vi "TrackingHelp.vi"() -> ()   [LabVIEW 2014]
panel:
  out "String":string="This mode is intended for tracking operation. Currently this mode works as a setpoint switcher where the ROV moves to the next WayPoint (WP) in the list when the current is reached. \n\nThe waypoint list will auto-index itself when entering new waypoints and is inserted automatically in the map view.\n\nIt is not possible to enter negative depth (height above the surface as ROVs cannot fly..yet).\n\nThe Generate Pattern Button opens a dialog box where inputs can be given in order to generate a lawn mower pattern. \n\nThe Read and Write WP buttons import and export the waypoints in their own file format: *.wp\n\nThe clear WP List button removes all the waypoints from the list, and also from the map."
  out "2D Picture":picture
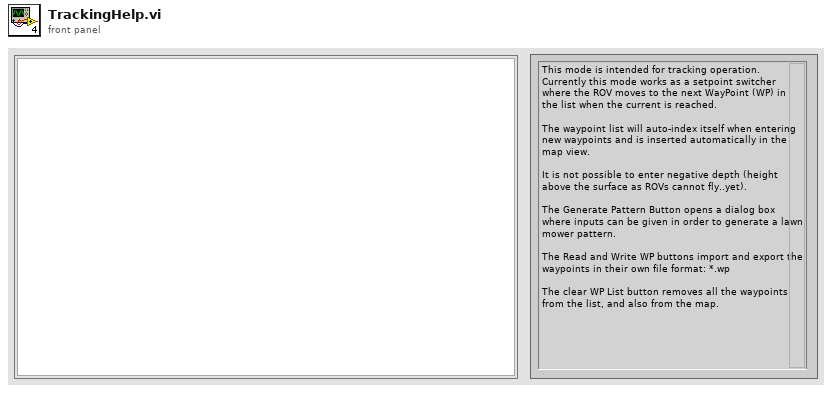
[diagram p1: front panel]
types:
  T1 = typedef "imagedata.ctl" = cluster{"image type":i32, "image depth":i32, "image":u8[], "mask":u8[], "colors":u32[], "Rectangle":cluster{"left":i16, "top":i16, "right":i16, "bottom":i16}}
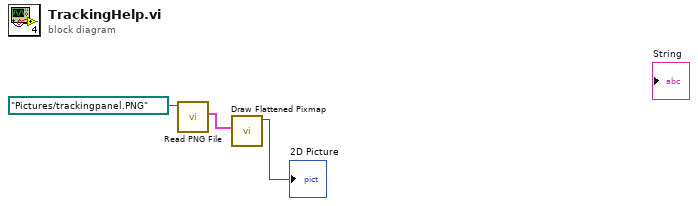
[diagram p0: block diagram]
diagram:
  n1 = call <vilib>:"Read PNG File.vi"("path to PNG file"=path "Pictures/trackingpanel.PNG") -> ("image data"=w2:T1)  [unwired: 8 in, 2 out]
  n2 = call <vilib>:"Draw Flattened Pixmap.vi"("image data"=w2) -> ("new picture"=→"2D Picture":picture)  [unwired: 8 in]
